vi "PowerOnAccess.vi"(0 "Operation Interface in":refnum<class "Operation Interface.lvclass">, 1 "Robot Status":T1, 5 "error in (no error)":errorcluster) -> (14 "Operation Interface out":refnum<class "Operation Interface.lvclass">, 15 "Robot Status Out":T1, 19 "error out":errorcluster)   [LabVIEW 2016, in "Operation Interface.lvclass"]
uses:
  Operation Interface.lvclass
  Universal Robot/RobotStatus.ctl
  Universal Robot/RobotMode.ctl
  Universal Robot/OperationalMode.ctl
  Universal Robot/SafetyStatus.ctl
  Operation Interface.lvclass/Operation Interface.ctl
  Universal Robot/Universal Robot.lvclass
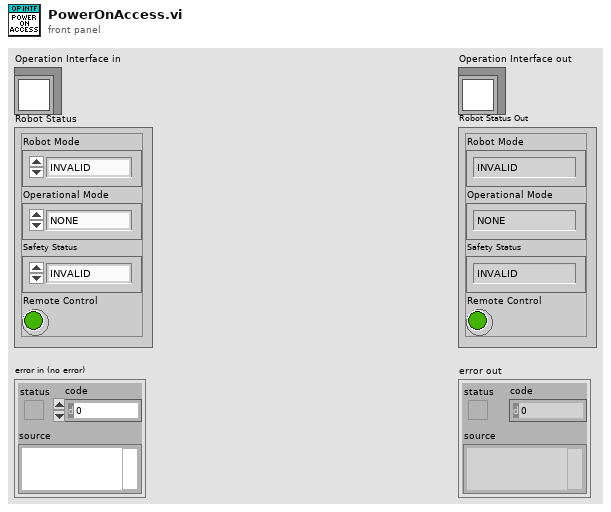
[diagram p1: front panel]
types:
  T1 = typedef "Universal Robot.lvclass/RobotStatus.ctl" = cluster{"Robot Mode":T2, "Operational Mode":T3, "Safety Status":T4, "Remote Control":bool}
  T2 = typedef "Universal Robot.lvclass/RobotMode.ctl" = enum16{"INVALID", "NO_CONTROLLER", "DISCONNECTED", "CONFIRM_SAFETY", "BOOTING", "POWER_OFF", "POWER_ON", "IDLE", "BACKDRIVE", "RUNNING"}
  T3 = typedef "Universal Robot.lvclass/OperationalMode.ctl" = enum16{"NONE", "MANUAL", "AUTOMATIC"}
  T4 = typedef "Universal Robot.lvclass/SafetyStatus.ctl" = enum16{"INVALID", "NORMAL", "REDUCED", "PROTECTIVE_STOP", "RECOVERY", "SAFEGAURD_STOP", "SYSTEM_EMERGENCY_STOP", "ROBOT_EMERGENCY_STOP", "VIOLATION", "FAULT", "AUTOMATIC_MODE_SAFEGAURD_STOP", "SYSTEM_THREE_POSITION_ENABLING_STOP"}
  T5 = enum8{"Enabled", "Disabled", "Disabled and Grayed Out"}
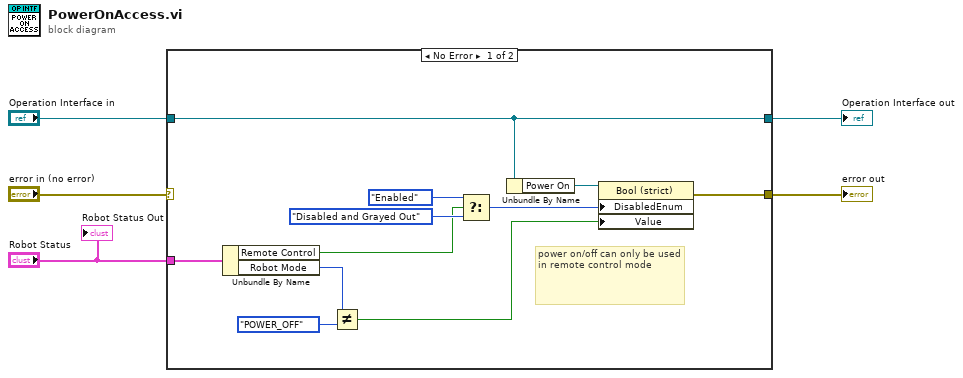
[diagram p0: block diagram]
diagram:
  n1 = case shown="No Error" "error in (no error)" {
    selector: "error in (no error)" -> [_ w18]
    tunnel: [w8 w18] -> w4
    tunnel: [w16 w17] -> w2
    tunnel: "Operation Interface in" -> [w16 w17]
    tunnel: "Robot Status" -> [w15 _]
    frame No Error {
      # "power on/off can only be used in remote control mode"
      n2 = Unbundle By Name(w15) -> ("Remote Control"=w6:bool, "Robot Mode"=w10:T2)
      n3 = Not Equal?(x=w10, y=RobotMode."POWER_OFF" ("x")) -> (x != y?=w7:bool)
      n4 = Select(t=T5."Enabled" ("Disabled"), s=w6, f=T5."Disabled and Grayed Out" ("Disabled")) -> (s? t:f=w9:T5)
      n5 = Unbundle By Name(w16) -> ("Power On"=w12:refnum<vi>)
      n6 = property class="Bool (strict)"(reference=w12, "DisabledEnum"=w9, "Value"=w7) -> (error out=w8:errorcluster)  [unwired: 1 in, 1 out]
    }
    frame Error {
    }
  }
  "error out" <- w4
  "Operation Interface out" <- w2
  "Robot Status Out" <- "Robot Status"
